vi "Correlation Coefficient (Kendall's Tau).vi"(10 "Y":dbl[](array[numeric]) format="%.2f", 11 "X":dbl[](array[numeric]) format="%.2f") -> (2 "r^2":dbl format="%.7g", 3 "correlation coefficient r":dbl format="%.7g")   [LabVIEW 2014, in "NI_Gmath.lvlib"]
doc: "Computes the Kendall's Tau correlation coefficient between input sequences <B>X</B> and <B>Y</B>."
uses:
  NI_Gmath.lvlib
panel:
  # "Correlation Coefficient \n(Kendall's Tau)"
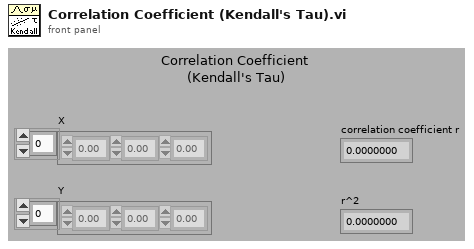
[diagram p1: front panel]
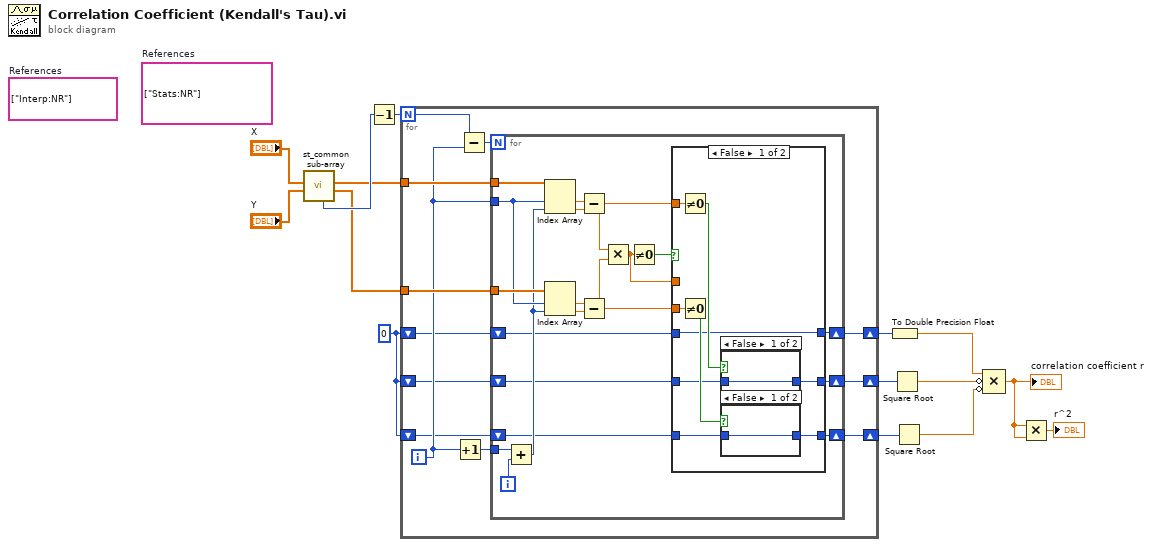
[diagram p0: block diagram]
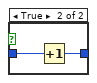
[diagram p2: hidden frame]
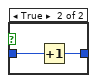
[diagram p3: hidden frame]
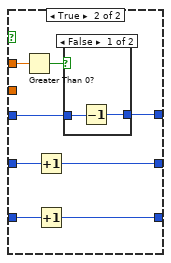
[diagram p4: hidden frame]
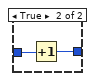
[diagram p5: hidden frame]
diagram:
  (unwired) string[] ["Stats:NR"]  # References
  w9 = 0
  (unwired) string[] ["Interp:NR"]  # References
  n1 = call "st_common sub-array.vi"(9:"array 1 in"="Y", 10:"array 1 in"="X") -> (1:"array 1 out"=w11:dbl[], 2:"array 1 out"=w12:dbl[], "size"=w13:i32)  [unwired: 7 in]
  n2 = Decrement(x=w13) -> (x-1=w10:i32)
  n3 = for {
    N: w10 -> [w26]
    tunnel: w12 -> [w25]
    tunnel: w11 -> [w24]
    shift-right: [w20] -> w8
    shift-left: w9 -> [w21]
    shift-right: [w18] -> w7
    shift-left: w9 -> [w19]
    shift-right: [w16] -> w6
    shift-left: w9 -> [w17]
    i -> [w23]
    n4 = Increment(x=w23) -> (x+1=w22:i32)
    n5 = Subtract(x=w26, y=w23) -> (x-y=w27:i32)
    n6 = for {
      N: w27 -> [_]
      tunnel: w25 -> [w47]
      tunnel: w24 -> [w44]
      tunnel: w23 -> [w43]
      tunnel: w22 -> [w45]
      shift-right: [w35] -> w20
      shift-left: w21 -> [w36]
      shift-right: [w33] -> w18
      shift-left: w19 -> [w34]
      shift-right: [w30] -> w16
      shift-left: w17 -> [w31]
      i -> [w46]
      n7 = Add(x=w45, y=w46) -> (x+y=w42:i32)
      n8 = Index Array(array=w47, index #1=w43, index #2=w42) -> (element #1=w41:dbl, element #2=w40:dbl)
      n9 = Index Array(array=w44, index #1=w43, index #2=w42) -> (element #1=w39:dbl, element #2=w38:dbl)
      n10 = Subtract(x=w41, y=w40) -> (x-y=w29:dbl)
      n11 = Subtract(x=w39, y=w38) -> (x-y=w28:dbl)
      n12 = Multiply(x=w29, y=w28) -> (x*y=w32:dbl)
      n13 = Not Equal To 0?(x=w32) -> (x != 0?=w37:bool)
      n14 = case shown="False" w37 {
        tunnel: w36 -> [w52 w70]
        tunnel: [w50 w69] -> w35
        tunnel: w34 -> [w51 w68]
        tunnel: [w49 w67] -> w33
        tunnel: w32 -> [_ w66]
        tunnel: w31 -> [w48 w64]
        tunnel: [w48 w63] -> w30
        tunnel: w29 -> [w56 _]
        tunnel: w28 -> [w55 _]
        frame False {
          n15 = Not Equal To 0?(x=w56) -> (x != 0?=w53:bool)
          n16 = Not Equal To 0?(x=w55) -> (x != 0?=w54:bool)
          n17 = case shown="False" w53 {
            tunnel: [w60 w62] -> w50
            tunnel: w52 -> [w60 w61]
            frame False {
            }
            frame True {
              n18 = Increment(x=w61) -> (x+1=w62:i32)
            }
          }
          n19 = case shown="False" w54 {
            tunnel: [w57 w59] -> w49
            tunnel: w51 -> [w57 w58]
            frame False {
            }
            frame True {
              n20 = Increment(x=w58) -> (x+1=w59:i32)
            }
          }
        }
        frame True {
          n21 = Greater Than 0?(x=w66) -> (x > 0?=w65:bool)
          n22 = Increment(x=w70) -> (x+1=w69:i32)
          n23 = Increment(x=w68) -> (x+1=w67:i32)
          n24 = case shown="False" w65 {
            tunnel: w64 -> [w72 w74]
            tunnel: [w71 w73] -> w63
            frame False {
              n25 = Decrement(x=w72) -> (x-1=w71:i32)
            }
            frame True {
              n26 = Increment(x=w74) -> (x+1=w73:i32)
            }
          }
        }
      }
    }
  }
  n27 = To Double Precision Float(number=w6) -> (double precision float=w5:dbl)
  n28 = Square Root(x=w8) -> (sqrt(x)=w4:dbl)
  n29 = Square Root(x=w7) -> (sqrt(x)=w3:dbl)
  n30 = Compound Arithmetic op=MULTIPLY(w5, invert w4, invert w3) -> (w1:dbl)
  "correlation coefficient r" <- w1
  n31 = Multiply(x=w1, y=w1) -> (x*y=→"r^2":dbl)
